vi "pyonpyon.vi"() -> ()   [LabVIEW 2013]
uses:
  <vilib>/DAQmx/create/channels.llb/DAQmx Create Channel (AO-Voltage-Basic).vi
  <vilib>/DAQmx/configure/timing.llb/DAQmx Timing (Sample Clock).vi
  <vilib>/DAQmx/create/channels.llb/DAQmx Create Channel (DO-Digital Output).vi
panel:
  in  "DAQmx Port -- Sound":tag="Dev2/ao0"
  in  "DAQmx Port  -- Trial Code":tag="Dev2/port0"
  in  "DAQmx Port -- Coulbourn Trig":tag="Dev2/port1"
  out "Session List/Total Trials Valid":bool=TRUE
  out "Trial Types Valid":bool=TRUE
  in  "Refresh":bool
  in  "Waveform Properties":T1={"Fs (Hz)"=20000.0, "Amplitude (V)"=1.0, "Ramp (s)"=0.005, "Duration (s)"=0.1} {"Ramp (s)" min=0.0; "Fs (Hz)" min=0.0}
  out "Current/Cued Trial":T2={"Trial Code"=2, "Trial Type"=enum."NOGO", "Trial Weight"=1, "Stim Type"=enum."FM Sweep", "Stim Dur (s)"=0.25, "Stim P1"=4000.0, "Stim P2"=2000.0} {"Stim P2" min=0.0; "Trial Weight" step=1; "Stim P1" min=0.0; "Stim Dur (s)" min=0.0; "Trial Code" min=1 step=1}
  in  "Default Trial":T2={"Trial Code"=1, "Trial Type"=enum."GO", "Trial Weight"=1, "Stim Type"=enum."FM Sweep", "Stim Dur (s)"=0.25, "Stim P1"=2000.0, "Stim P2"=4000.0} {"Stim P2" min=0.0; "Trial Weight" step=1; "Stim P1" min=0.0; "Stim Dur (s)" min=0.0; "Trial Code" min=1 step=1}
  in  "Add Trial":bool
  in  "Trial Types":T3(array[cluster])=[{"Trial Code"=1, "Trial Type"=enum."GO", "Trial Weight"=1, "Stim Type"=enum."FM Sweep", "Stim Dur (s)"=0.25, "Stim P1"=2000.0, "Stim P2"=4000.0}, {"Trial Code"=2, "Trial Type"=enum."NOGO", "Trial Weight"=1, "Stim Type"=enum."FM Sweep", "Stim Dur (s)"=0.25, "Stim P1"=4000.0, "Stim P2"=2000.0}] {"Stim P2" min=0.0; "Trial Weight" step=1; "Stim P1" min=0.0; "Stim Dur (s)" min=0.0; "Trial Code" min=1 step=1}
  in  "Initial Intertrial":dbl=180.0 caption="Initial Intertrial (s)\n(Habituation--only valid for Trial #0)"
  in  "Intertrial Upper Bound":dbl=30.0 caption="Intertrial Upper Bound (s)"
  in  "Intertrial Lower Bound":dbl=20.0 caption="Intertrial Lower Bound (s)"
  in  "stop":bool
  in  "Save Session List":bool
  out "Runtime Errors":errorcluster
  out "Current (or Cued) Waveform":waveform(dbl)(graph)={"t0"=timestamp(0 s since 1904-01-01), "dt"=5e-05, "Y"=array[5000 elements]}
  out "Playing Stimulus":bool caption="Playing stimulus"
  in  "Current (or Cued) Trial":i32(slide)=100 max=10 scale=0.0..99.0
  out "Waiting for trigger":bool
  out "Session List File Path":path=path "E:/Data/SPP.Coulb1/SPP022/ppSessList.140903.1454.tsv"
  in  "Load Session List":bool
  out "Trial Types File Path":path
  in  "Load Trial Types":bool
  in  "Save Trial Types":bool
  in  "Total Trials":i32=100 min=3 step=1
  out "Session List (Cannot Edit)":i32[](array[numeric])=[1, 1, 2, 2, 2, 1, 2, 1, 2, 1, 1, 2, 1, 1, 2, 2, 1, 2, 1, 2, 2, 2, 1, 1, 2, 1, 2, 1, 2, 1, 2, 1, 1, 1, 2, 2, 1, 2, 1, 2, 1, 2, 1, 2, 1, 2, 1, 2, 1, 1, 1, 2, 1, 1, 1, 2, 1, 1, 2, 1, 2, 2, 1, 2, 1, 2, 2, 2, 1, 2, 1, 2, 2, 1, 2, 2, 1, 2, 1, 1, 1, 2, 2, 2, 1, 1, 2, 2, 2, 1, 2, 1, 1, 1, 2, 2, 1, 1, 2, 2]
  in  "Play Session  List":bool
  in  "Generate Session List":bool
  # "Default Trial to Add"
  # "Trial Code"
  # "Trial Type"
  # "Trial Wt"
  # "Stim Type"
  # "Stim Dur (s)"
  # "Stim P1"
  # "Stim P2"
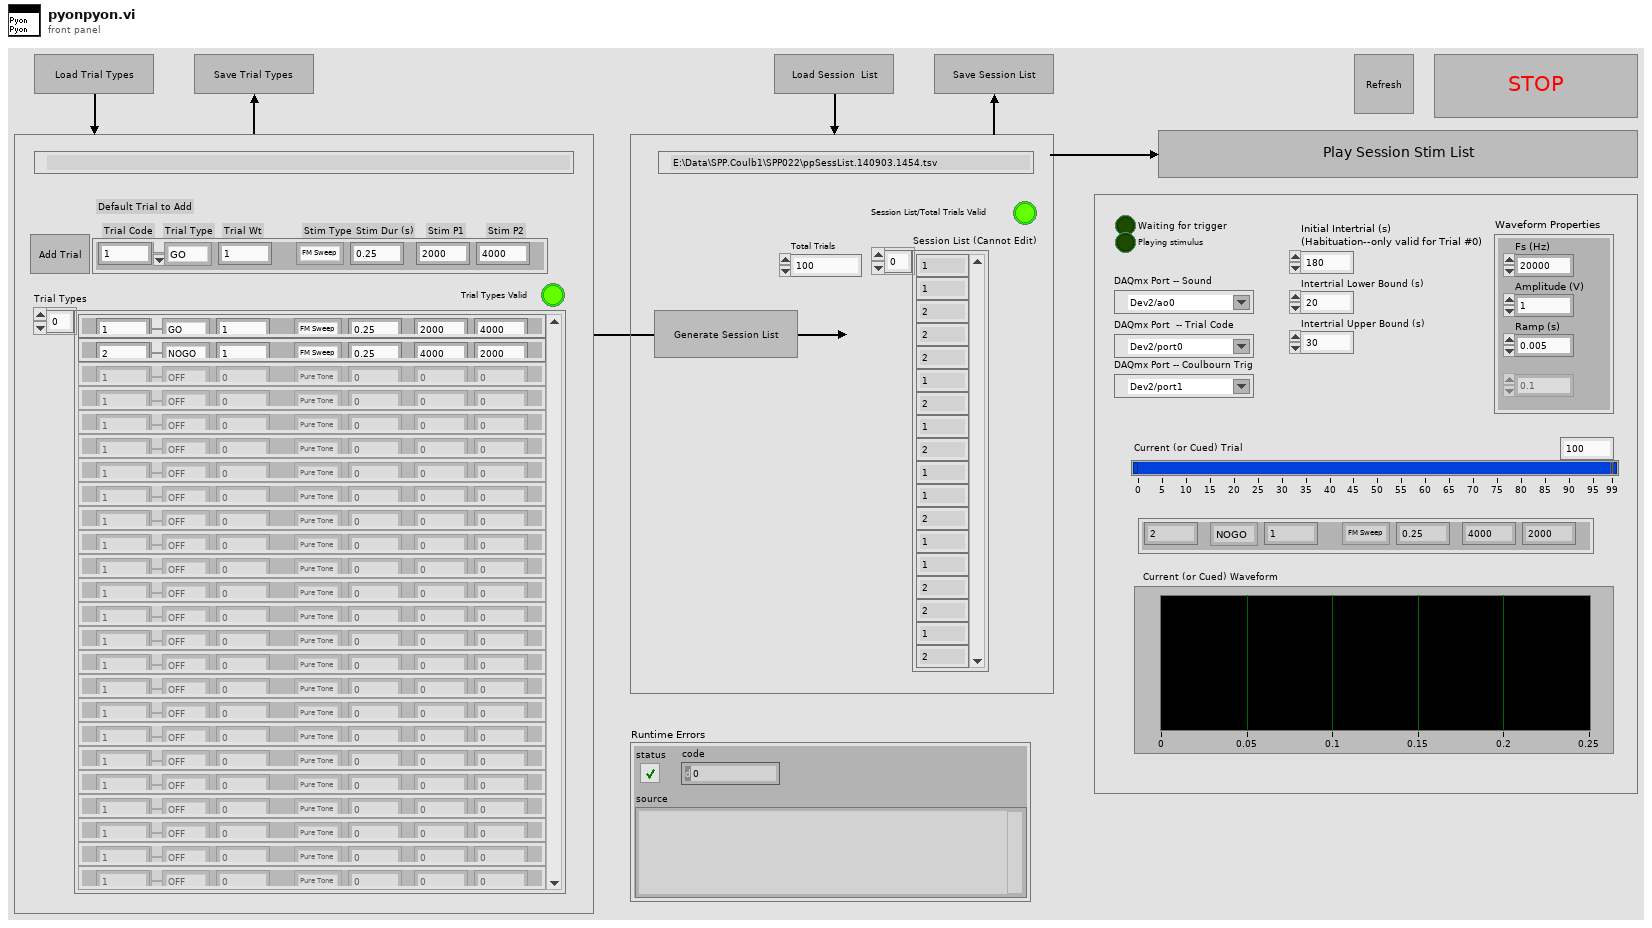
[diagram p1: front panel]
types:
  T1 = cluster{"Fs (Hz)":dbl, "Amplitude (V)":dbl, "Ramp (s)":dbl, "Duration (s)":dbl}
  T2 = cluster{"Trial Code":u16, "Trial Type":enum16{"OFF", "GO", "NOGO", "TEST"}, "Trial Weight":u32, "Stim Type":enum16{"Pure Tone", "FM Sweep"}, "Stim Dur (s)":dbl, "Stim P1":dbl, "Stim P2":dbl}
  T3 = cluster{"Trial Code":u16, "Trial Type":enum16{"OFF", "GO", "NOGO", "TEST"}, "Trial Weight":u32, "Stim Type":enum16{"Pure Tone", "FM Sweep"}, "Stim Dur (s)":dbl, "Stim P1":dbl, "Stim P2":dbl}[]
  T4 = enum8{"Enabled", "Disabled", "Disabled and Grayed Out"}
  T5 = cluster{u16, "Trial Type":enum16{"OFF", "GO", "NOGO", "TEST"}, "Trial Weight":u32, "Stim Type":enum16{"Pure Tone", "FM Sweep"}, "Stim Dur (s)":dbl, "Stim P1":dbl, "Stim P2":dbl}
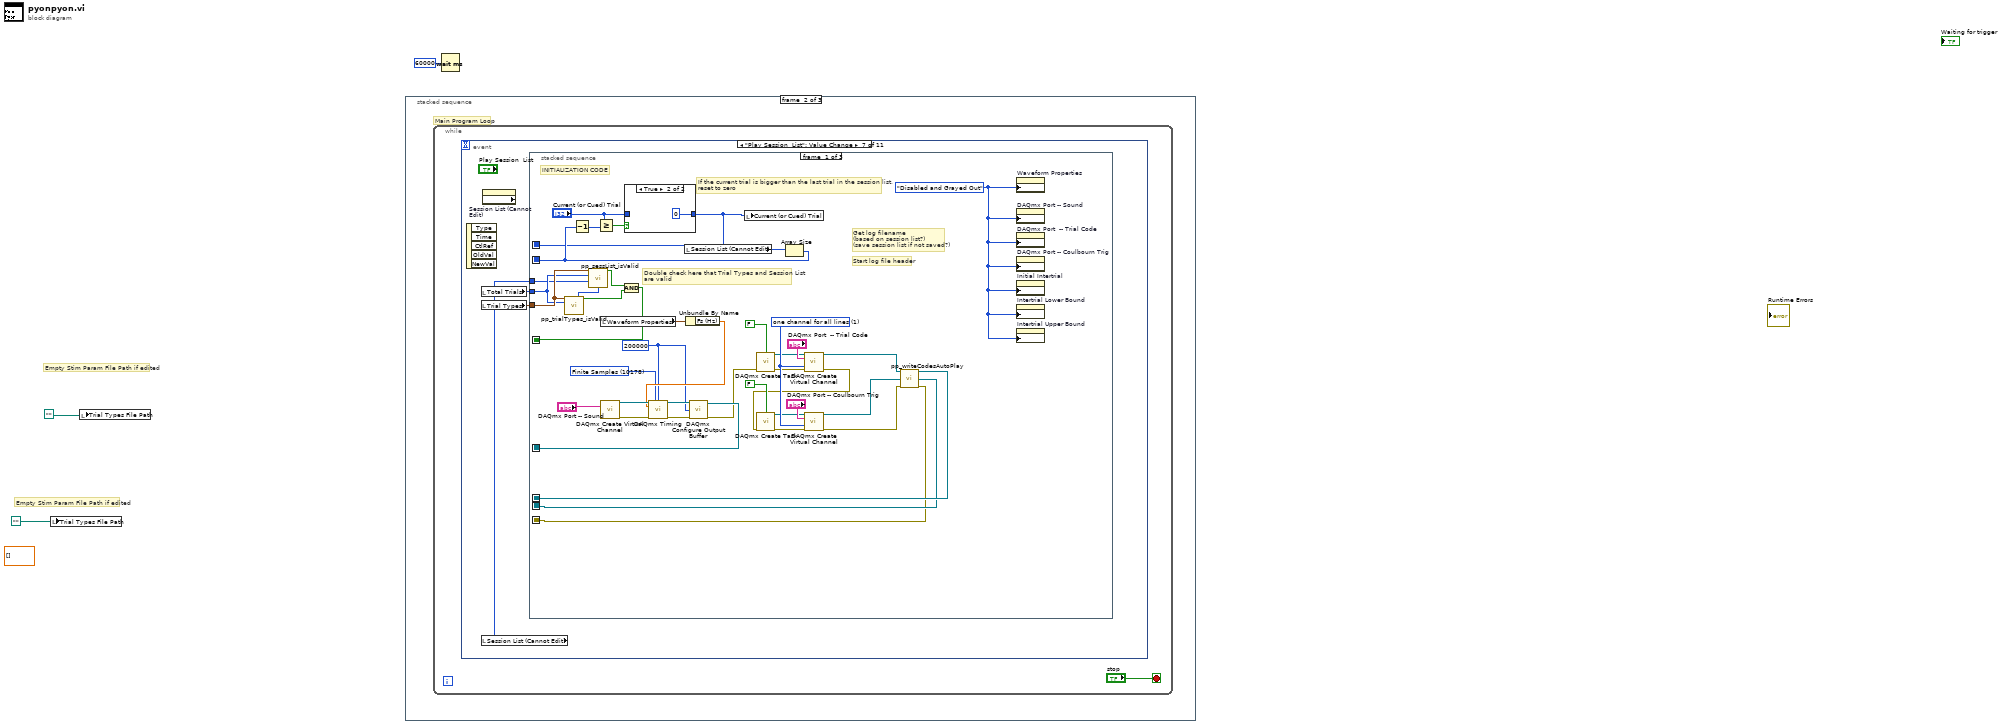
[diagram p0: block diagram]
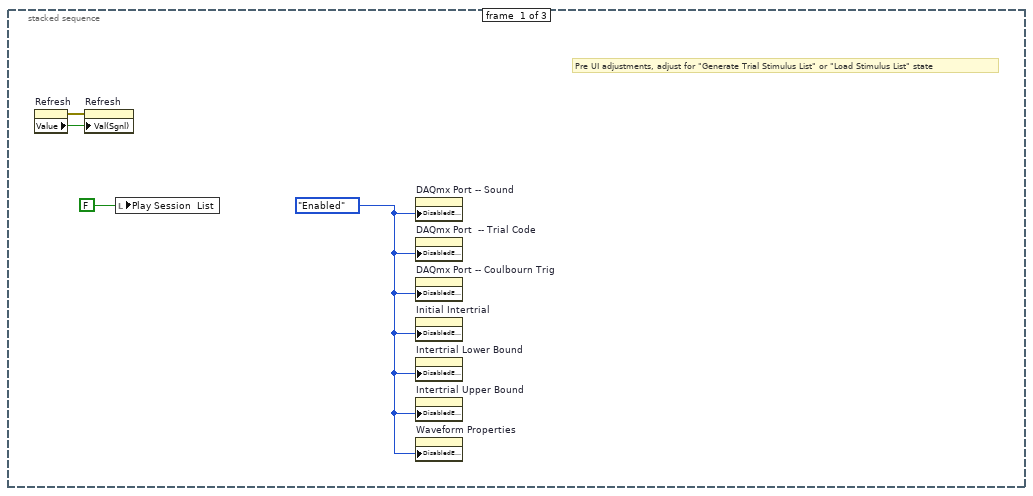
[diagram p2: hidden frame]
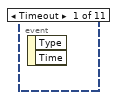
[diagram p3: hidden frame]
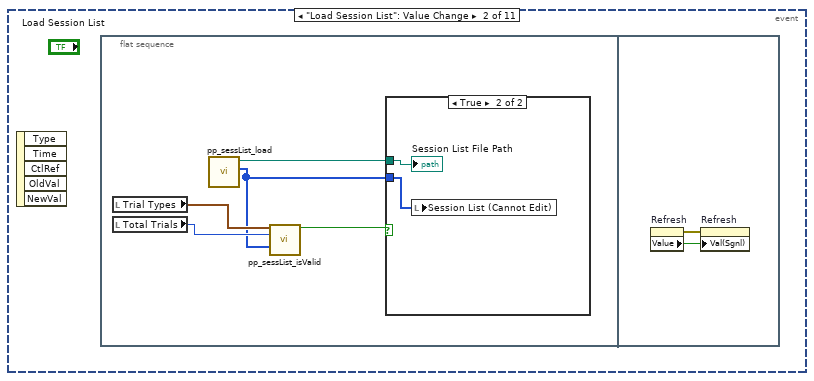
[diagram p4: hidden frame]
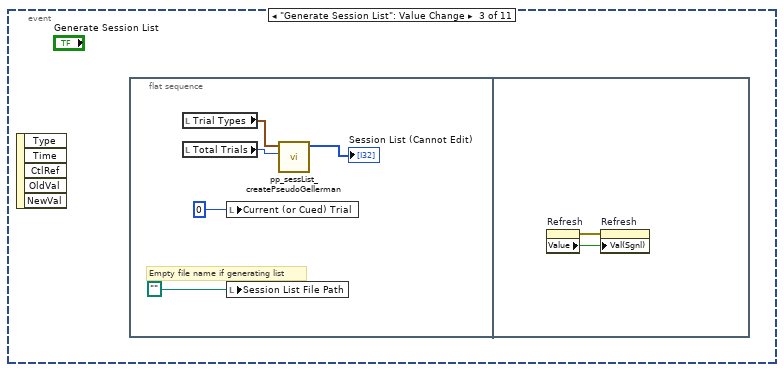
[diagram p6: hidden frame]
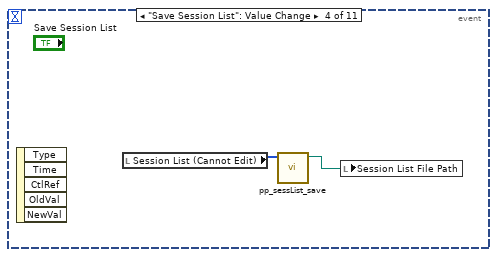
[diagram p7: hidden frame]
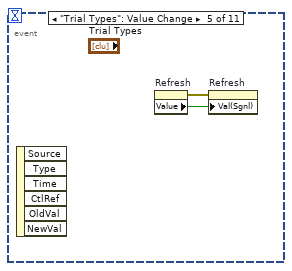
[diagram p8: hidden frame]
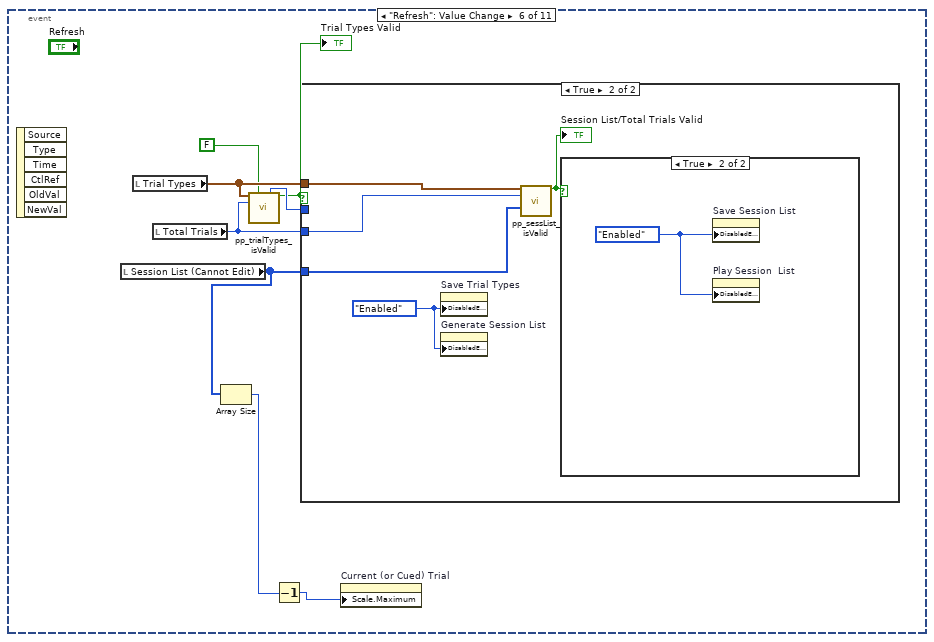
[diagram p9: hidden frame]
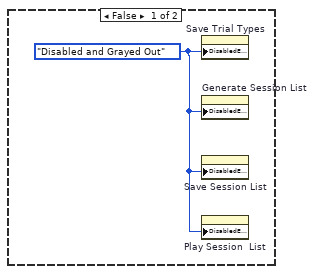
[diagram p10: hidden frame]
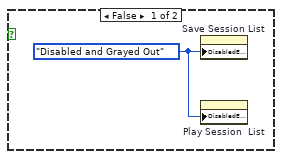
[diagram p11: hidden frame]
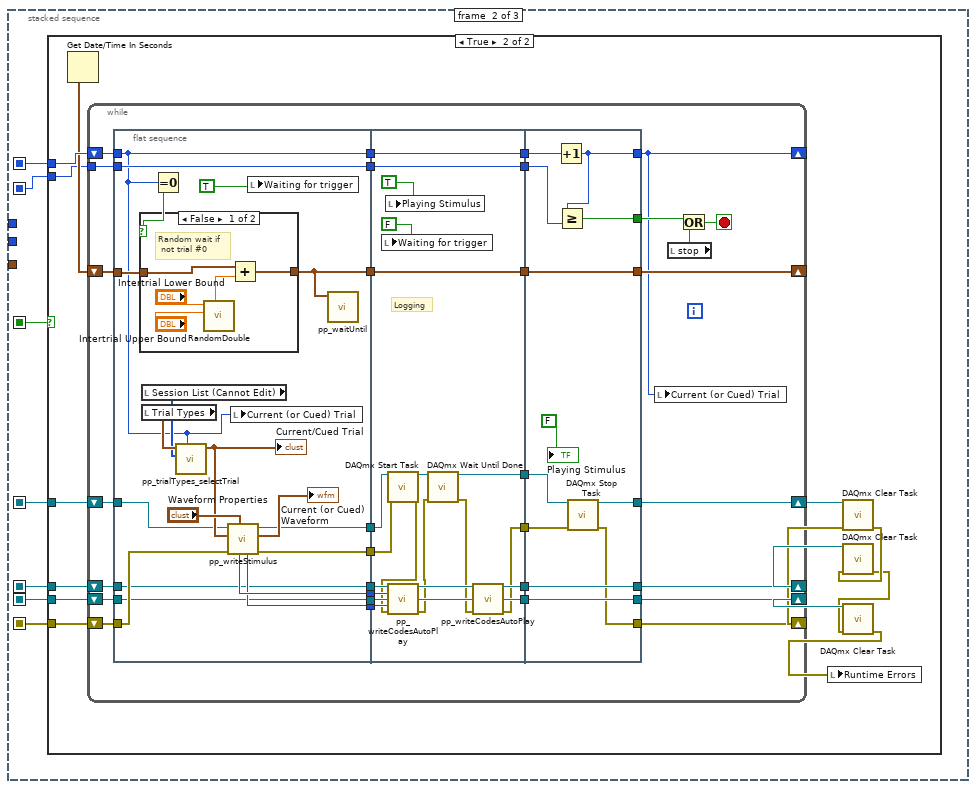
[diagram p13: hidden frame]
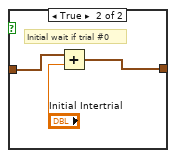
[diagram p15: hidden frame]
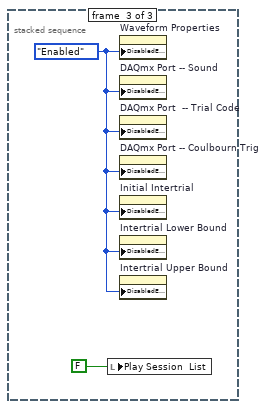
[diagram p16: hidden frame]
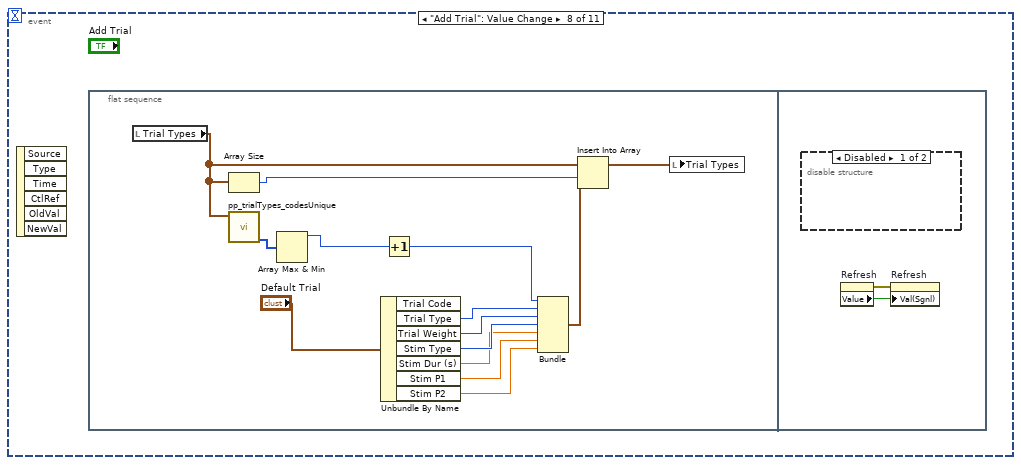
[diagram p17: hidden frame]
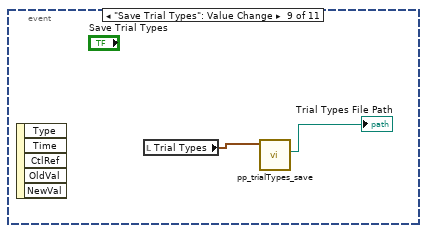
[diagram p19: hidden frame]
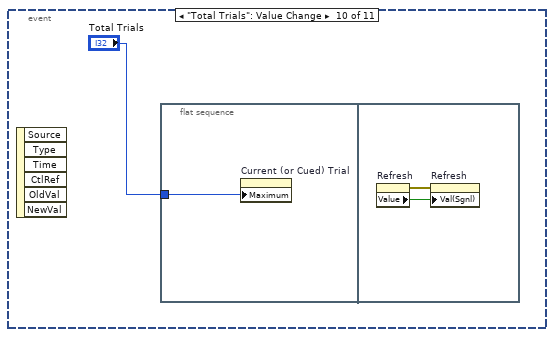
[diagram p20: hidden frame]
diagram:
  (unwired) dbl[][] []
  # "Empty Stim Param File Path if edited"
  # "Empty Stim Param File Path if edited"
  n1 = local write "Trial Types File Path"(path "") -> ()
  n2 = local write "Trial Types File Path"(path "") -> ()
  n3 = stacked-sequence {
    frame #0 {
      w4 = T4."Enabled" ("Disabled")
      # "Pre UI adjustments, adjust for \"Generate Trial Stimulus List\" or \"Load Stimulus List\" state"
      n4 = property on="Refresh" class="Bool (strict)"() -> (error out=w7:errorcluster, "Value"=w6:bool)  [unwired: 2 in, 1 out]
      n5 = property on="Refresh" class="Bool (strict)"(error in=w7, "Val(Sgnl)"=w6) -> ()  [unwired: 1 in, 2 out]
      n6 = local write "Play Session  List"(FALSE ("Play Session  List")) -> ()
      n7 = property on="DAQmx Port -- Sound" class="DAQmxName"("DisabledEnum"=w4) -> ()  [unwired: 2 in, 2 out]
      n8 = property on="DAQmx Port  -- Trial Code" class="DAQmxName"("DisabledEnum"=w4) -> ()  [unwired: 2 in, 2 out]
      n9 = property on="DAQmx Port -- Coulbourn Trig" class="DAQmxName"("DisabledEnum"=w4) -> ()  [unwired: 2 in, 2 out]
      n10 = property on="Initial Intertrial" class="DigNum (strict)"("DisabledEnum"=w4) -> ()  [unwired: 2 in, 2 out]
      n11 = property on="Intertrial Lower Bound" class="DigNum (strict)"("DisabledEnum"=w4) -> ()  [unwired: 2 in, 2 out]
      n12 = property on="Intertrial Upper Bound" class="DigNum (strict)"("DisabledEnum"=w4) -> ()  [unwired: 2 in, 2 out]
      n13 = property on="Waveform Properties" class="Clust (strict)"("DisabledEnum"=w4) -> ()  [unwired: 2 in, 2 out]
    }
    frame #1 {
      # "Main Program Loop"
      n14 = while {
        stop <- "stop" stop-if-true
        n15 = event shown="[6] \"Play Session  List\": Value Change" {
          selector: _ -> [_ _ _ _ _ _ _ _ _ _ _]
          dyn-events: _ -> [_ _ _ _ _ _ _ _ _ _ _]
          timeout: _ -> [_ _ _ _ _ _ _ _ _ _ _]
          event Timeout {
            n16 = event-data() -> ()  [unwired: 1 in, 2 out]
          }
          event "Load Session List": Value Change {
            n17 = event-data() -> ()  [unwired: 1 in, 5 out]
            n18 = flat-sequence {
              frame #0 {
                n19 = local read "Trial Types"() -> (w12:T3)
                n20 = local read "Total Trials"() -> (w11:i32)
                n21 = call "pp_sessList_load.vi"() -> ("Session List (Cannot Edit)"=w9:i32[], "Session List File Path"=w10:path)  [unwired: 9 in, 1 out]
                n22 = call "pp_sessList_isValid.vi"("Trial Types"=w12, "Total Trials"=w11, "Session List"=w9) -> ("Session List Valid?"=w13:bool)  [unwired: 12 in]
                n23 = case shown="True" w13 {
                  tunnel: w10 -> [_ w14]
                  tunnel: w9 -> [_ w15]
                  frame False {
                  }
                  frame True {
                    n24 = local write "Session List (Cannot Edit)"(w15) -> ()
                    "Session List File Path" <- w14
                  }
                }
              }
              frame #1 {
                n25 = property on="Refresh" class="Bool (strict)"() -> (error out=w17:errorcluster, "Value"=w16:bool)  [unwired: 2 in, 1 out]
                n26 = property on="Refresh" class="Bool (strict)"(error in=w17, "Val(Sgnl)"=w16) -> ()  [unwired: 1 in, 2 out]
              }
            }
          }
          event "Generate Session List": Value Change {
            n27 = event-data() -> ()  [unwired: 1 in, 5 out]
            n28 = flat-sequence {
              frame #0 {
                # "Empty file name if generating list"
                n29 = local read "Trial Types"() -> (w19:T3)
                n30 = local read "Total Trials"() -> (w20:i32)
                n31 = local write "Current (or Cued) Trial"(0 ("Current (or Cued) Trial")) -> ()
                n32 = local write "Session List File Path"(path "") -> ()
                n33 = call "pp_sessList_createPseudoGellerman.vi"("Total Trials"=w20, "Trial Types"=w19) -> ("Session List (Cannot Edit)"=→"Session List (Cannot Edit)":i32[])  [unwired: 8 in, 1 out]
              }
              frame #1 {
                n34 = property on="Refresh" class="Bool (strict)"() -> (error out=w24:errorcluster, "Value"=w23:bool)  [unwired: 2 in, 1 out]
                n35 = property on="Refresh" class="Bool (strict)"(error in=w24, "Val(Sgnl)"=w23) -> ()  [unwired: 1 in, 2 out]
              }
            }
          }
          event "Save Session List": Value Change {
            n36 = event-data() -> ()  [unwired: 1 in, 5 out]
            n37 = local read "Session List (Cannot Edit)"() -> (w25:i32[])
            n38 = call "pp_sessList_save.vi"("Session List (Cannot Edit)"=w25) -> ("Session List File Path"=w26:path)  [unwired: 9 in, 1 out]
            n39 = local write "Session List File Path"(w26) -> ()
          }
          event "Trial Types": Value Change {
            n40 = event-data() -> ()  [unwired: 1 in, 6 out]
            n41 = property on="Refresh" class="Bool (strict)"() -> (error out=w27:errorcluster, "Value"=w28:bool)  [unwired: 2 in, 1 out]
            n42 = property on="Refresh" class="Bool (strict)"(error in=w27, "Val(Sgnl)"=w28) -> ()  [unwired: 1 in, 2 out]
          }
          event "Refresh": Value Change {
            n43 = event-data() -> ()  [unwired: 1 in, 6 out]
            n44 = local read "Session List (Cannot Edit)"() -> (w31:i32[])
            n45 = local read "Trial Types"() -> (w34:T3)
            n46 = local read "Total Trials"() -> (w35:i32)
            n47 = Array Size(array=w31) -> (size(s)=w30:i32)
            n48 = call "pp_trialTypes_isValid.vi"("Trial Types"=w34, "Throw Error"=FALSE, "Total Trials"=w35) -> ("Trial Replication Factor"=w36:i32, "Paradigm Valid?"=w32:bool)  [unwired: 7 in, 4 out]
            "Trial Types Valid" <- w32
            n49 = Decrement(x=w30) -> (x-1=w29:i32)
            n50 = case shown="True" w32 {
              tunnel: w34 -> [_ w42]
              tunnel: w36 -> [_ _]
              tunnel: w35 -> [_ w41]
              tunnel: w31 -> [_ w38]
              frame False {
                w37 = T4."Disabled and Grayed Out" ("Disabled")
                n51 = property on="Save Trial Types" class="Bool"("DisabledEnum"=w37) -> ()  [unwired: 2 in, 2 out]
                n52 = property on="Generate Session List" class="Bool"("DisabledEnum"=w37) -> ()  [unwired: 2 in, 2 out]
                n53 = property on="Save Session List" class="Bool"("DisabledEnum"=w37) -> ()  [unwired: 2 in, 2 out]
                n54 = property on="Play Session  List" class="Bool (strict)"("DisabledEnum"=w37) -> ()  [unwired: 2 in, 2 out]
              }
              frame True {
                w40 = T4."Enabled" ("Disabled")
                n55 = property on="Save Trial Types" class="Bool"("DisabledEnum"=w40) -> ()  [unwired: 2 in, 2 out]
                n56 = property on="Generate Session List" class="Bool"("DisabledEnum"=w40) -> ()  [unwired: 2 in, 2 out]
                n57 = call "pp_sessList_isValid.vi"("Trial Types"=w42, "Total Trials"=w41, "Session List"=w38) -> ("Session List Valid?"=w39:bool)  [unwired: 12 in]
                "Session List/Total Trials Valid" <- w39
                n58 = case shown="True" w39 {
                  frame False {
                    w43 = T4."Disabled and Grayed Out" ("Disabled")
                    n59 = property on="Save Session List" class="Bool"("DisabledEnum"=w43) -> ()  [unwired: 2 in, 2 out]
                    n60 = property on="Play Session  List" class="Bool (strict)"("DisabledEnum"=w43) -> ()  [unwired: 2 in, 2 out]
                  }
                  frame True {
                    w44 = T4."Enabled" ("Disabled")
                    n61 = property on="Save Session List" class="Bool"("DisabledEnum"=w44) -> ()  [unwired: 2 in, 2 out]
                    n62 = property on="Play Session  List" class="Bool (strict)"("DisabledEnum"=w44) -> ()  [unwired: 2 in, 2 out]
                  }
                }
              }
            }
            n63 = property on="Current (or Cued) Trial" class="Slide (strict)"("Scale.Maximum"=w29) -> ()  [unwired: 2 in, 2 out]
          }
          event "Play Session  List": Value Change {
            n64 = event-data() -> ()  [unwired: 1 in, 5 out]
            n65 = local read "Total Trials"() -> (w45:i32)
            n66 = local read "Trial Types"() -> (w47:T3)
            n67 = local read "Session List (Cannot Edit)"() -> (w46:i32[])
            n68 = property on="Session List (Cannot Edit)" class="Arr (strict)" props=["Number of Rows"]() -> ()  [unwired: 2 in, 3 out]
            n69 = stacked-sequence {
              seq-local: [w77 _ _] -> [_ w97 _]
              seq-local: [w55 _ _] -> [_ w95 _]
              seq-local: [w54 _ _] -> [_ w96 _]
              seq-local: [w56 _ _] -> [_ w92 _]
              seq-local: [w50 _ _] -> [_ w94 _]
              seq-local: [w80 _ _] -> [_ w93 _]
              seq-local: [w51 _ _] -> [_ w91 _]
              tunnel: w47 -> [w85 _ _]
              tunnel: w46 -> [w83 _ _]
              tunnel: w45 -> [w84 _ _]
              frame #0 {
                w49 = 10178 items=["Finite Samples"=10178, "Continuous Samples"=10123, "Hardware Timed Single Point"=12522] ("sample mode")
                w72 = T4."Disabled and Grayed Out" ("Disabled")
                w48 = u32 200000 ("Input.BufSize")
                w69 = 1 items=["one channel for each line", "one channel for all lines"] ("line grouping")
                # "Double check here that Trial Types and Session List\nare valid"
                # "If the current trial is bigger than the last trial in the session list, \nreset to zero"
                # "INITIALIZATION CODE"
                # "Start log file header"
                # "Get log filename\n(based on session list?)\n(save session list if not saved?)"
                n70 = call "pp_trialTypes_isValid.vi"("Trial Types"=w85, "Total Trials"=w84) -> ("Trial Replication Factor"=w86:i32, "Paradigm Valid?"=w81:bool)  [unwired: 8 in, 4 out]
                n71 = call "pp_sessList_isValid.vi"("Trial Types"=w85, "Total Trials"=w84, "Session List"=w83, "Trial Replication Factor"=w86) -> ("Session List Valid?"=w82:bool)  [unwired: 11 in]
                n72 = local read "Waveform Properties"() -> (w71:T1)
                n73 = call-poly <vilib>:"DAQmx Create Virtual Channel.vi"("physical channels"="DAQmx Port -- Sound") -> ("task out"=w76:refnum<k21>, "error out"=w73:errorcluster)  [unwired: 13 in]
                n74 = And(x=w82, y=w81) -> (x .and. y?=w80:bool)
                n75 = local read "Session List (Cannot Edit)"() -> (w53:i32[])
                n76 = Unbundle By Name(w71) -> ("Fs (Hz)"=w70:dbl)
                n77 = call-poly <vilib>:"DAQmx Timing.vi"("task/channels in"=w76, "sample mode"=w49, "samples per channel"=w48, "rate"=w70, "error in"=w73) -> ("task out"=w75:refnum<k21>, "error out"=w74:errorcluster)  [unwired: 9 in]
                n78 = call <vilib>:"DAQmx Configure Output Buffer.vi"("task/channels in"=w75, "buffer size (in samples per channel)"=w48, "error in"=w74) -> ("task out"=w77:refnum<k21>, "error out"=w64:errorcluster)  [unwired: 11 in]
                n79 = call <vilib>:"DAQmx Create Task.vi"("auto cleanup"=FALSE, "error in"=w64) -> ("task out"=w63:refnum<k21>, "error out"=w65:errorcluster)  [unwired: 12 in]
                n80 = Array Size(array=w53) -> (size(s)=w51:i32)
                n81 = Decrement(x=w51) -> (x-1=w52:i32)
                n82 = Greater Or Equal?(x="Current (or Cued) Trial", y=w52) -> (x >= y?=w88:bool)
                n83 = case shown="True" w88 {
                  tunnel: "Current (or Cued) Trial" -> [w89 _]
                  tunnel: [w89 0] -> w50
                  frame False {
                  }
                  frame True {
                  }
                }
                n84 = local write "Current (or Cued) Trial"(w50) -> ()
                n85 = call-poly <vilib>:"DAQmx Create Virtual Channel.vi"("task in"=w63, "lines"="DAQmx Port  -- Trial Code", "line grouping"=w69, "error in"=w65) -> ("task out"=w59:refnum<k21>, "error out"=w60:errorcluster)  [unwired: 10 in]
                n86 = call <vilib>:"DAQmx Create Task.vi"("auto cleanup"=FALSE, "error in"=w60) -> ("task out"=w66:refnum<k21>, "error out"=w67:errorcluster)  [unwired: 12 in]
                n87 = call-poly <vilib>:"DAQmx Create Virtual Channel.vi"("task in"=w66, "lines"="DAQmx Port -- Coulbourn Trig", "line grouping"=w69, "error in"=w67) -> ("task out"=w58:refnum<k21>, "error out"=w57:errorcluster)  [unwired: 10 in]
                n88 = call "pp_writeCodesAutoPlay.vi"("DAQmx Digital Out 1 In"=w59, "DAQmx Digital Out 2 In"=w58, "Error In"=w57) -> ("DAQmx Digital Out 1 Out"=w56:refnum<k21>, "DAQmx Digital Out 2 Out"=w55:refnum<k21>, "Error Out"=w54:errorcluster)  [unwired: 10 in]
                n89 = property on="Waveform Properties" class="Clust (strict)"("DisabledEnum"=w72) -> ()  [unwired: 2 in, 2 out]
                n90 = property on="DAQmx Port -- Sound" class="DAQmxName"("DisabledEnum"=w72) -> ()  [unwired: 2 in, 2 out]
                n91 = property on="DAQmx Port  -- Trial Code" class="DAQmxName"("DisabledEnum"=w72) -> ()  [unwired: 2 in, 2 out]
                n92 = property on="DAQmx Port -- Coulbourn Trig" class="DAQmxName"("DisabledEnum"=w72) -> ()  [unwired: 2 in, 2 out]
                n93 = property on="Initial Intertrial" class="DigNum (strict)"("DisabledEnum"=w72) -> ()  [unwired: 2 in, 2 out]
                n94 = property on="Intertrial Lower Bound" class="DigNum (strict)"("DisabledEnum"=w72) -> ()  [unwired: 2 in, 2 out]
                n95 = property on="Intertrial Upper Bound" class="DigNum (strict)"("DisabledEnum"=w72) -> ()  [unwired: 2 in, 2 out]
              }
              frame #1 {
                n96 = case shown="True" w93 {
                  tunnel: w97 -> [_ w111]
                  tunnel: w96 -> [_ w110]
                  tunnel: w94 -> [_ w109]
                  tunnel: w95 -> [_ w108]
                  tunnel: w91 -> [_ w106]
                  tunnel: w92 -> [_ w104]
                  frame False {
                  }
                  frame True {
                    n97 = Get Date/Time In Seconds() -> (seconds since 1Jan1904=w107:timestamp)
                    n98 = while {
                      shift-right: [w113] -> w102
                      shift-left: w108 -> [w143]
                      shift-right: [w138] -> w105
                      shift-left: w111 -> [w142]
                      shift-right: [w112] -> _
                      shift-left: w109 -> [w141]
                      shift-right: [w116] -> w101
                      shift-left: w110 -> [w139]
                      shift-right: [w130] -> _
                      shift-left: w107 -> [w133]
                      tunnel: w106 -> [w129]
                      shift-right: [w114] -> w103
                      shift-left: w104 -> [w125]
                      stop <- w135 stop-if-true
                      n99 = flat-sequence {
                        tunnel: w143 -> [w145]
                        tunnel: w142 -> [w149]
                        tunnel: w141 -> [w155]
                        tunnel: [w155] -> w140
                        tunnel: w139 -> [w151]
                        tunnel: w133 -> [w160]
                        tunnel: [w157] -> w132
                        tunnel: w129 -> [w158]
                        tunnel: [w158] -> w127
                        tunnel: w125 -> [w146]
                        tunnel: [w152] -> w123
                        tunnel: [w148] -> w122
                        tunnel: [w147] -> w121
                        tunnel: [w146] -> w120
                        tunnel: [w145] -> w119
                        tunnel: [w144] -> w115
                        tunnel: w140 -> [w187]
                        tunnel: [w188] -> w137
                        tunnel: [w187] -> w136
                        tunnel: w132 -> [w186]
                        tunnel: [w186] -> w131
                        tunnel: [w185] -> w128
                        tunnel: w127 -> [w185]
                        tunnel: [w171] -> w124
                        tunnel: w123 -> [w184]
                        tunnel: w122 -> [w183]
                        tunnel: w121 -> [w182]
                        tunnel: w120 -> [w181]
                        tunnel: w119 -> [w180]
                        tunnel: [w177] -> w118
                        tunnel: [w176] -> w117
                        tunnel: w115 -> [w178]
                        tunnel: [w196] -> w138
                        tunnel: w137 -> [w197]
                        tunnel: w136 -> [w203]
                        tunnel: [w202] -> w126
                        tunnel: [w198] -> w112
                        tunnel: w131 -> [w201]
                        tunnel: [w201] -> w130
                        tunnel: w128 -> [w200]
                        tunnel: w124 -> [w195]
                        tunnel: w118 -> [w194]
                        tunnel: w117 -> [w193]
                        tunnel: [w192] -> w116
                        tunnel: [w194] -> w114
                        tunnel: [w193] -> w113
                        frame #0 {
                          n100 = local read "Session List (Cannot Edit)"() -> (w156:i32[])
                          n101 = local read "Trial Types"() -> (w159:T3)
                          n102 = Equal To 0?(x=w155) -> (x = 0?=w161:bool)
                          n103 = case shown="False" w161 {
                            tunnel: w160 -> [w163 w170]
                            tunnel: [w164 w168] -> w157
                            frame False {
                              # "Random wait if\n not trial #0"
                              n104 = call "RandomDouble.vi"("Min"="Intertrial Upper Bound", "Max"="Intertrial Lower Bound") -> ("Random"=w165:dbl)  [unwired: 9 in]
                              n105 = Add(x=w163, y=w165) -> (x+y=w164:timestamp)
                            }
                            frame True {
                              # "Initial wait if trial #0"
                              n106 = Add(x=w170, y="Initial Intertrial") -> (x+y=w168:timestamp)
                            }
                          }
                          n107 = call "pp_trialTypes_selectTrial.vi"("Current Session Trial"=w155, "Session List (Cannot Edit)"=w156, "Trial Types"=w159) -> ("Current/Cued Trial"=w150:T2)  [unwired: 7 in, 1 out]
                          "Current/Cued Trial" <- w150
                          n108 = call "pp_writeStimulus.vi"("Waveform Properties"="Waveform Properties", "Error In"=w151, "Current/Cued Trial"=w150, "DAQmx Analog Out In"=w149) -> ("Error Out"=w144:errorcluster, "Waveform Out"=→"Current (or Cued) Waveform":waveform(dbl), "DAQmx Analog Out Out"=w152:refnum<k21>, "Trial Type"=w147:u8, "Trial Code"=w148:u8)  [unwired: 3 in]
                          n109 = local write "Current (or Cued) Trial"(w155) -> ()
                          n110 = local write "Waiting for trigger"(TRUE) -> ()
                          n111 = call "pp_waitUntil.vi"("until time"=w157) -> ()  [unwired: 11 in]
                        }
                        frame #1 {
                          # "Logging"
                          n112 = local write "Waiting for trigger"(FALSE) -> ()
                          n113 = local write "Playing Stimulus"(TRUE) -> ()
                          n114 = call <vilib>:"DAQmx Start Task.vi"("task/channels in"=w184, "error in"=w178) -> ("task out"=w191:refnum<k21>, "error out"=w179:errorcluster)  [unwired: 12 in]
                          n115 = call "pp_writeCodesAutoPlay.vi"("DAQmx Digital Out 1 In"=w181, "Digital Out 1 Value"=w183, "DAQmx Digital Out 2 In"=w180, "Digital Out 2 Value"=w182, "Error In"=w179) -> ("DAQmx Digital Out 1 Out"=w175:refnum<k21>, "DAQmx Digital Out 2 Out"=w174:refnum<k21>, "Error Out"=w172:errorcluster)  [unwired: 8 in]
                          n116 = call <vilib>:"DAQmx Wait Until Done.vi"("task/channels in"=w191, "error in"=w172) -> ("task out"=w188:refnum<k21>, "error out"=w173:errorcluster)  [unwired: 12 in]
                          n117 = call "pp_writeCodesAutoPlay.vi"("DAQmx Digital Out 1 In"=w175, "DAQmx Digital Out 2 In"=w174, "Error In"=w173) -> ("DAQmx Digital Out 1 Out"=w177:refnum<k21>, "DAQmx Digital Out 2 Out"=w176:refnum<k21>, "Error Out"=w171:errorcluster)  [unwired: 10 in]
                        }
                        frame #2 {
                          n118 = Increment(x=w203) -> (x+1=w198:i32)
                          n119 = Greater Or Equal?(x=w198, y=w200) -> (x >= y?=w202:bool)
                          n120 = call <vilib>:"DAQmx Stop Task.vi"("task/channels in"=w197, "error in"=w195) -> ("task out"=w196:refnum<k21>, "error out"=w192:errorcluster)  [unwired: 12 in]
                          "Playing Stimulus" <- FALSE ("Playing Stimulus")
                        }
                      }
                      n121 = local write "Current (or Cued) Trial"(w112) -> ()
                      n122 = local read "stop"() -> (w134:bool)
                      n123 = Or(x=w126, y=w134) -> (x .or. y?=w135:bool)
                    }
                    n124 = call <vilib>:"DAQmx Clear Task.vi"("task in"=w105, "error in"=w101) -> ("error out"=w100:errorcluster)  [unwired: 13 in]
                    n125 = call <vilib>:"DAQmx Clear Task.vi"("task in"=w103, "error in"=w100) -> ("error out"=w99:errorcluster)  [unwired: 13 in]
                    n126 = call <vilib>:"DAQmx Clear Task.vi"("task in"=w102, "error in"=w99) -> ("error out"=w98:errorcluster)  [unwired: 13 in]
                    n127 = local write "Runtime Errors"(w98) -> ()
                  }
                }
              }
              frame #2 {
                w205 = T4."Enabled" ("Disabled")
                n128 = local write "Play Session  List"(FALSE ("Play Session  List")) -> ()
                n129 = property on="Waveform Properties" class="Clust (strict)"("DisabledEnum"=w205) -> ()  [unwired: 2 in, 2 out]
                n130 = property on="DAQmx Port -- Sound" class="DAQmxName"("DisabledEnum"=w205) -> ()  [unwired: 2 in, 2 out]
                n131 = property on="DAQmx Port  -- Trial Code" class="DAQmxName"("DisabledEnum"=w205) -> ()  [unwired: 2 in, 2 out]
                n132 = property on="DAQmx Port -- Coulbourn Trig" class="DAQmxName"("DisabledEnum"=w205) -> ()  [unwired: 2 in, 2 out]
                n133 = property on="Initial Intertrial" class="DigNum (strict)"("DisabledEnum"=w205) -> ()  [unwired: 2 in, 2 out]
                n134 = property on="Intertrial Lower Bound" class="DigNum (strict)"("DisabledEnum"=w205) -> ()  [unwired: 2 in, 2 out]
                n135 = property on="Intertrial Upper Bound" class="DigNum (strict)"("DisabledEnum"=w205) -> ()  [unwired: 2 in, 2 out]
              }
            }
          }
          event "Add Trial": Value Change {
            n136 = event-data() -> ()  [unwired: 1 in, 6 out]
            n137 = flat-sequence {
              frame #0 {
                n138 = local read "Trial Types"() -> (w206:T3)
                n139 = Array Size(array=w206) -> (size(s)=w207:i32)
                n140 = call "pp_trialTypes_codesUnique.vi"("Trial Types"=w206) -> ("Code List"=w211:u16[])  [unwired: 9 in, 1 out]
                n141 = Array Max & Min(array=w211) -> (max value=w210:u16)  [unwired: 3 out]
                n142 = Unbundle By Name("Default Trial") -> ("Trial Type"=w217:enum16{"OFF", "GO", "NOGO", "TEST"}, "Trial Weight"=w216:u32, "Stim Type"=w215:enum16{"Pure Tone", "FM Sweep"}, "Stim Dur (s)"=w214:dbl, "Stim P1"=w213:dbl, "Stim P2"=w212:dbl)  [unwired: 1 out]
                n143 = Increment(x=w210) -> (x+1=w209:u16)
                n144 = Bundle(w209, "Trial Type"=w217, "Trial Weight"=w216, "Stim Type"=w215, "Stim Dur (s)"=w214, "Stim P1"=w213, "Stim P2"=w212) -> (w208:T5)  [unwired: 1 in]
                n145 = Insert Into Array(array=w206, index=w207, new element=w208) -> (w219:T3)
                n146 = local write "Trial Types"(w219) -> ()
              }
              frame #1 {
                n147 = disable-structure shown="Disabled" {
                  frame Disabled {
                  }
                  frame Enabled {
                  }
                }
                n148 = property on="Refresh" class="Bool (strict)"() -> (error out=w220:errorcluster, "Value"=w221:bool)  [unwired: 2 in, 1 out]
                n149 = property on="Refresh" class="Bool (strict)"(error in=w220, "Val(Sgnl)"=w221) -> ()  [unwired: 1 in, 2 out]
              }
            }
          }
          event "Save Trial Types": Value Change {
            n150 = event-data() -> ()  [unwired: 1 in, 5 out]
            n151 = local read "Trial Types"() -> (w223:T3)
            n152 = call "pp_trialTypes_save.vi"("Trial Types"=w223) -> ("Path"=→"Trial Types File Path":path)  [unwired: 9 in, 1 out]
          }
          event "Total Trials": Value Change {
            n153 = event-data() -> ()  [unwired: 1 in, 6 out]
            n154 = flat-sequence {
              tunnel: "Total Trials" -> [w225]
              frame #0 {
                n155 = property on="Current (or Cued) Trial" class="Slide (strict)"("Maximum"=w225) -> ()  [unwired: 2 in, 2 out]
              }
              frame #1 {
                n156 = property on="Refresh" class="Bool (strict)"() -> (error out=w226:errorcluster, "Value"=w227:bool)  [unwired: 2 in, 1 out]
                n157 = property on="Refresh" class="Bool (strict)"(error in=w226, "Val(Sgnl)"=w227) -> ()  [unwired: 1 in, 2 out]
              }
            }
          }
          event "Load Trial Types": Value Change {
            n158 = event-data() -> ()  [unwired: 1 in, 5 out]
            n159 = flat-sequence {
              frame #0 {
                n160 = call "pp_trialTypes_load.vi"() -> ("Path"=w228:path, "Trial Types"=w229:T3)  [unwired: 5 in, 1 out]
                n161 = local write "Trial Types File Path"(w228) -> ()
                n162 = local write "Trial Types"(w229) -> ()
              }
              frame #1 {
                n163 = property on="Refresh" class="Bool (strict)"() -> (error out=w231:errorcluster, "Value"=w230:bool)  [unwired: 2 in, 1 out]
                n164 = property on="Refresh" class="Bool (strict)"(error in=w231, "Val(Sgnl)"=w230) -> ()  [unwired: 1 in, 2 out]
              }
            }
          }
        }
      }
    }
    frame #2 {
      # "Post UI Adjustments"
      n165 = local write "stop"(FALSE ("stop")) -> ()
      n166 = local write "Play Session  List"(FALSE ("Play Session  List")) -> ()
    }
  }
  n167 = Wait (ms)(milliseconds to wait=u32 60000) -> ()  [unwired: 1 out]
